vi "Main.vi"() -> ()   [LabVIEW 2017]
doc: "This VI was generated automatically using the FPGA Wizard. You can modify the VI normally."
uses:
  <vilib>/rvi/interface/nirviMethod/nirviMethod.xnode
  <vilib>/rvi/interface/nirviCloseFPGA/nirviCloseFPGA.xnode
  <vilib>/rvi/interface/nirviOpenFPGA/nirviOpenFPGA.xnode
  <vilib>/rvi/interface/nirviReadWriteControl/nirviReadWriteControl.xnode
  <vilib>/rvi/errors/niLvFpgaAdjustHostInterfaceError.vi
  <vilib>/rvi/interface/Simulation/niFpgaSimulationCallBeginRW.vi
  <vilib>/FPGAPlugInAG/Dynamic/niLvFpga_ReadFifo_Dynamic.vi
  <vilib>/rvi/errors/niLvFpgaMergeErrorWithErrorCode.vi
  HostCode.lvlib
  <vilib>/Utility/file.llb/Write To Spreadsheet File (I64).vi
  <vilib>/Utility/error.llb/Error Cluster From Error Code.vi
  NiFpgaLv.dll
  SerialComm/SerialComm.lvclass
  C:/Program Files (x86)/National Instruments/LabVIEW 2017/examples/Instrument IO/Serial/support/Serial - Settings.ctl
  <vilib>/FPGAPlugInAG/Dynamic/niLvFpga_Reset_Dynamic.vi
  <vilib>/FPGAPlugInAG/Dynamic/niLvFpga_Run_Dynamic.vi
  FPGA Bitfiles/ECGPWMAdaptiveFi_FPGATarget2_ECGAFSPIInput_AXfYGaptw90old.lvbitx
  <vilib>/FPGAPlugInAG/Dynamic/niLvFpga_Close_Dynamic.vi
  <vilib>/FPGAPlugInAG/USB-7856R/niLvFpga_Open_USB-7856R.vi
  <vilib>/rvi/interface/common/dynamic/niFpgaDynamicAddResources.vi
  FPGACode/Lead Enum.ctl
  Trigger Params.ctl
  FPGACode/Channel Enum.ctl
panel:
  in  "Beta":u8(slide)=1 scale=0.0..3.0
  in  "Sensis\nECG Scaling":i16=1 caption="ECG Output\nScaling" min=1 max=100 step=1
  in  "Tab Control":enum32{"Main", "Utilities"}(tab)
  out "ECG":i16[][](graph)
  out "Invasive Blood Pressure":i16[][](graph)
  in  "Trigger 2":T1={"Channel"=enum."II", "Threshold"=1000, "d/dt"=FALSE, "Invert"=FALSE}
  out "Trigger":i16[][](graph)
  in  "IBP Scale":fxp<+/-,16,5>=1.06005859375
  in  "IBP Offset":fxp<+/-,16,16>
  in  "IBP Filter":bool
  in  "ECG Filter":bool=TRUE
  in  "Plot Info":T4={"Element"={"Lead"=enum."I", "Filter"=TRUE}, "Element 2"={"Lead"=enum."II", "Filter"=TRUE}, "Element 3"={"Lead"=enum."III", "Filter"=TRUE}}
  out "Pressure Data":T5(array[cluster])
  out "Gradients":i16[][](graph)
  in  "Offset":cluster{"X":i16, "Y":i16, "Z":i16} {"Z" format="%.2f"; "Y" format="%.2f"; "X" format="%.2f"}
  in  "High Pass Filter":bool
  out "Taps":dbl[](graph)
  out "Weights":dbl[](graph)
  out "Beta Product":fxp<+/-,32,-1> format="%.3e"
  out "Weighted Sum":fxp<+/-,33,19> format="%.3e"
  in  "Channel":i32
  in  "ECG Input\nGain":u16(ring)=1 items=["1"=1, "2"=2, "3"=3, "4"=4, "6"=0, "8"=5, "12"=6]
  in  "ECG Beta":fxp<+/-,32,-16>=1.000088900582341e-11 format="%.3e"
  in  "Filter Size":i16=100
  in  "IBP Beta":fxp<+/-,32,-16> format="%.3e"
  in  "Record":bool
  in  "Path":path
  out "Loop Time":u32
  in  "Reset":bool
  out "Actual Loop Rate (Ticks)":u32
  out "Late? Latched":bool
  in  "Start":bool
  in  "Loop Rate (Hz)":dbl=10000.0
  out "Calculated Rate (Hz)":dbl
  out "error out":errorcluster
  in  "Global Stop":bool
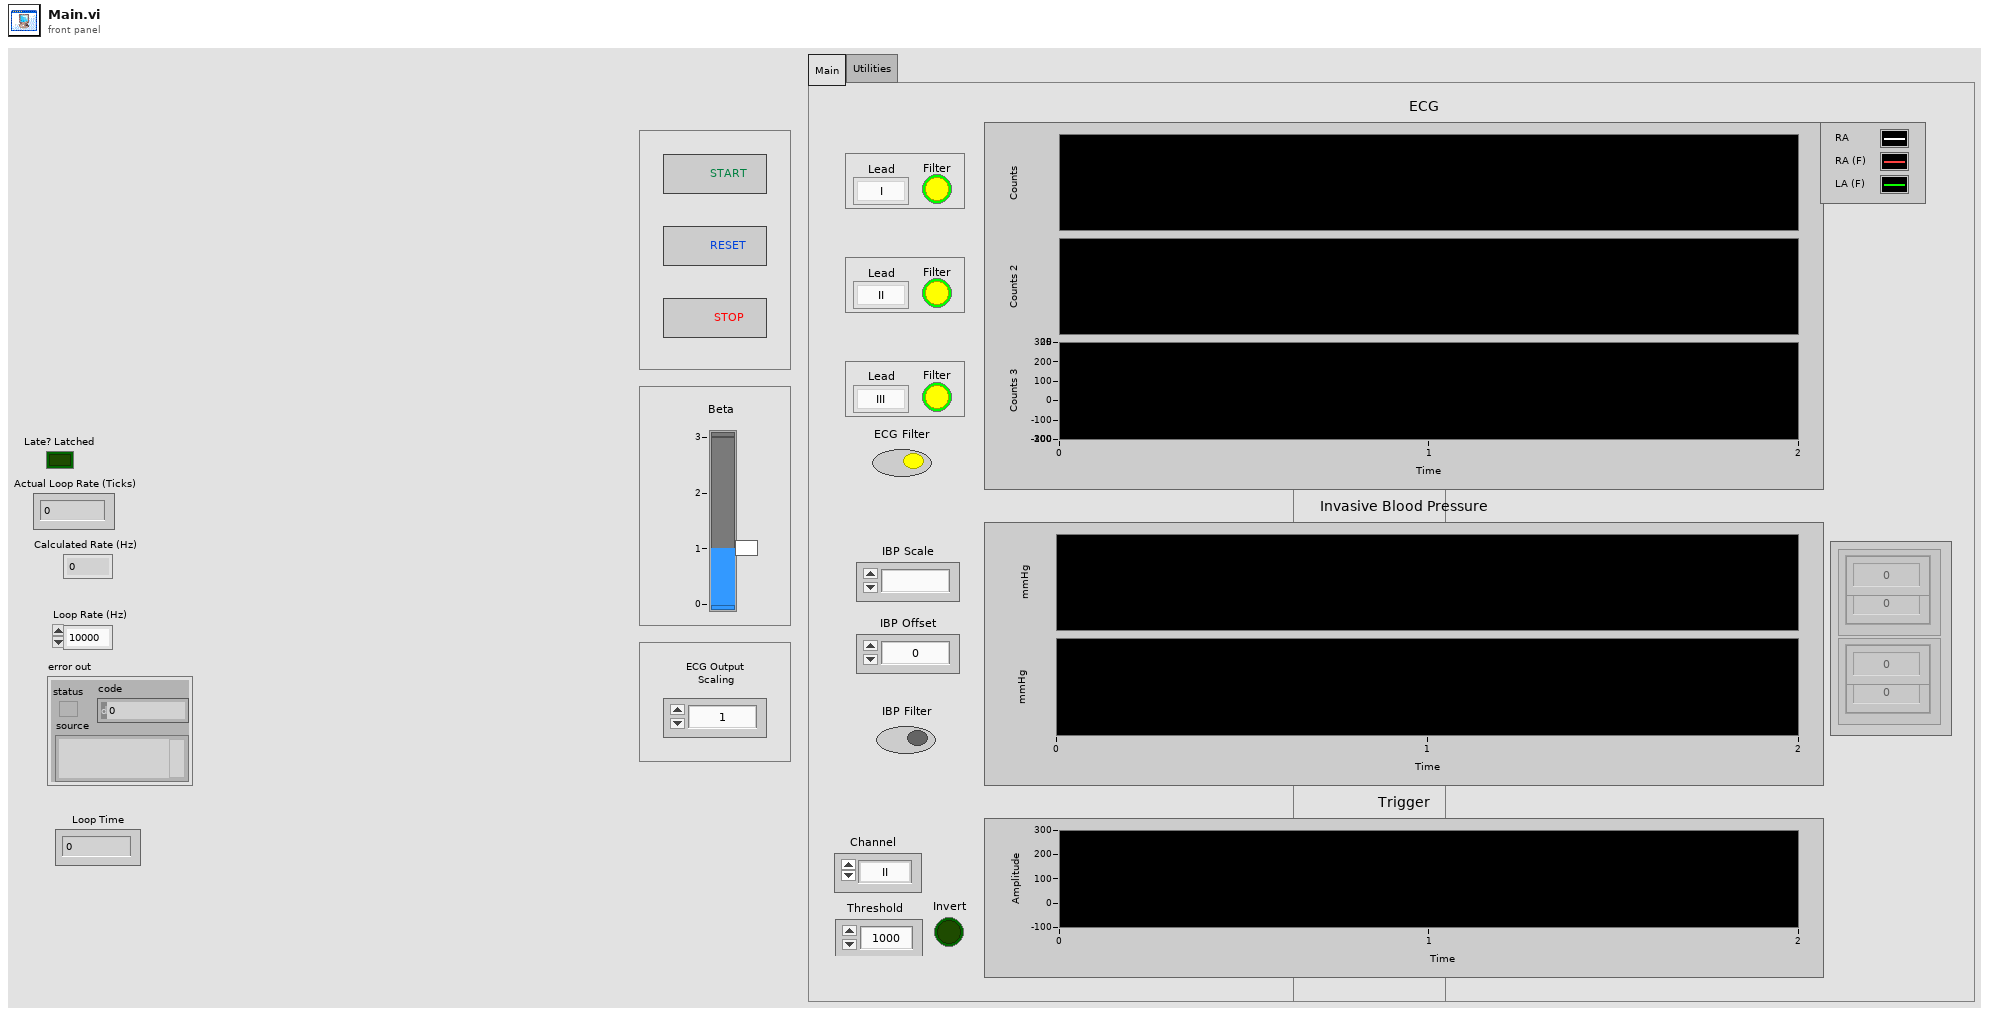
[diagram p1: front panel]
types:
  T1 = typedef "HostCode.lvlib/Trigger Params.ctl" = cluster{"Channel":T2, "Threshold":i16, "d/dt":bool, "Invert":bool}
  T2 = typedef "Channel Enum.ctl" = enum16{"RA", "LA", "LL", "V1", "V2", "V3", "V4", "V5", "V6", "I", "II", "III", "aVR", "aVL", "aVF", "Vw", "IBP1", "IBP2"}
  T3 = typedef "Lead Enum.ctl" = enum16{"RA", "LA", "LL", "V1", "V2", "V3", "V4", "V5", "V6", "I", "II", "III", "aVR", "aVL", "aVF", "Vw"}
  T4 = cluster{"Element":cluster{"Lead":T3, "Filter":bool}, "Element 2":cluster{"Lead":T3, "Filter":bool}, "Element 3":cluster{"Lead":T3, "Filter":bool}}
  T5 = cluster{"Numeric Control":dbl, "Numeric Control":dbl}[]
  T6 = typedef "Serial - Settings.ctl" = cluster{"baud rate":u32, "data bits":u16, "parity":enum16{"None", "Odd", "Even", "Mark", "Space"}, "stop bits":u16, "flow control":u16}
  T7 = enum8{"Enabled", "Disabled", "Disabled and Grayed Out"}
  T8 = typedef "LVOffsetAndMultiplierTypeDef.ctl" = cluster{"Offset":dbl, "Multiplier":dbl}
  T9 = cluster{"Channel":T2, "Threshold":i16, "Invert":bool}
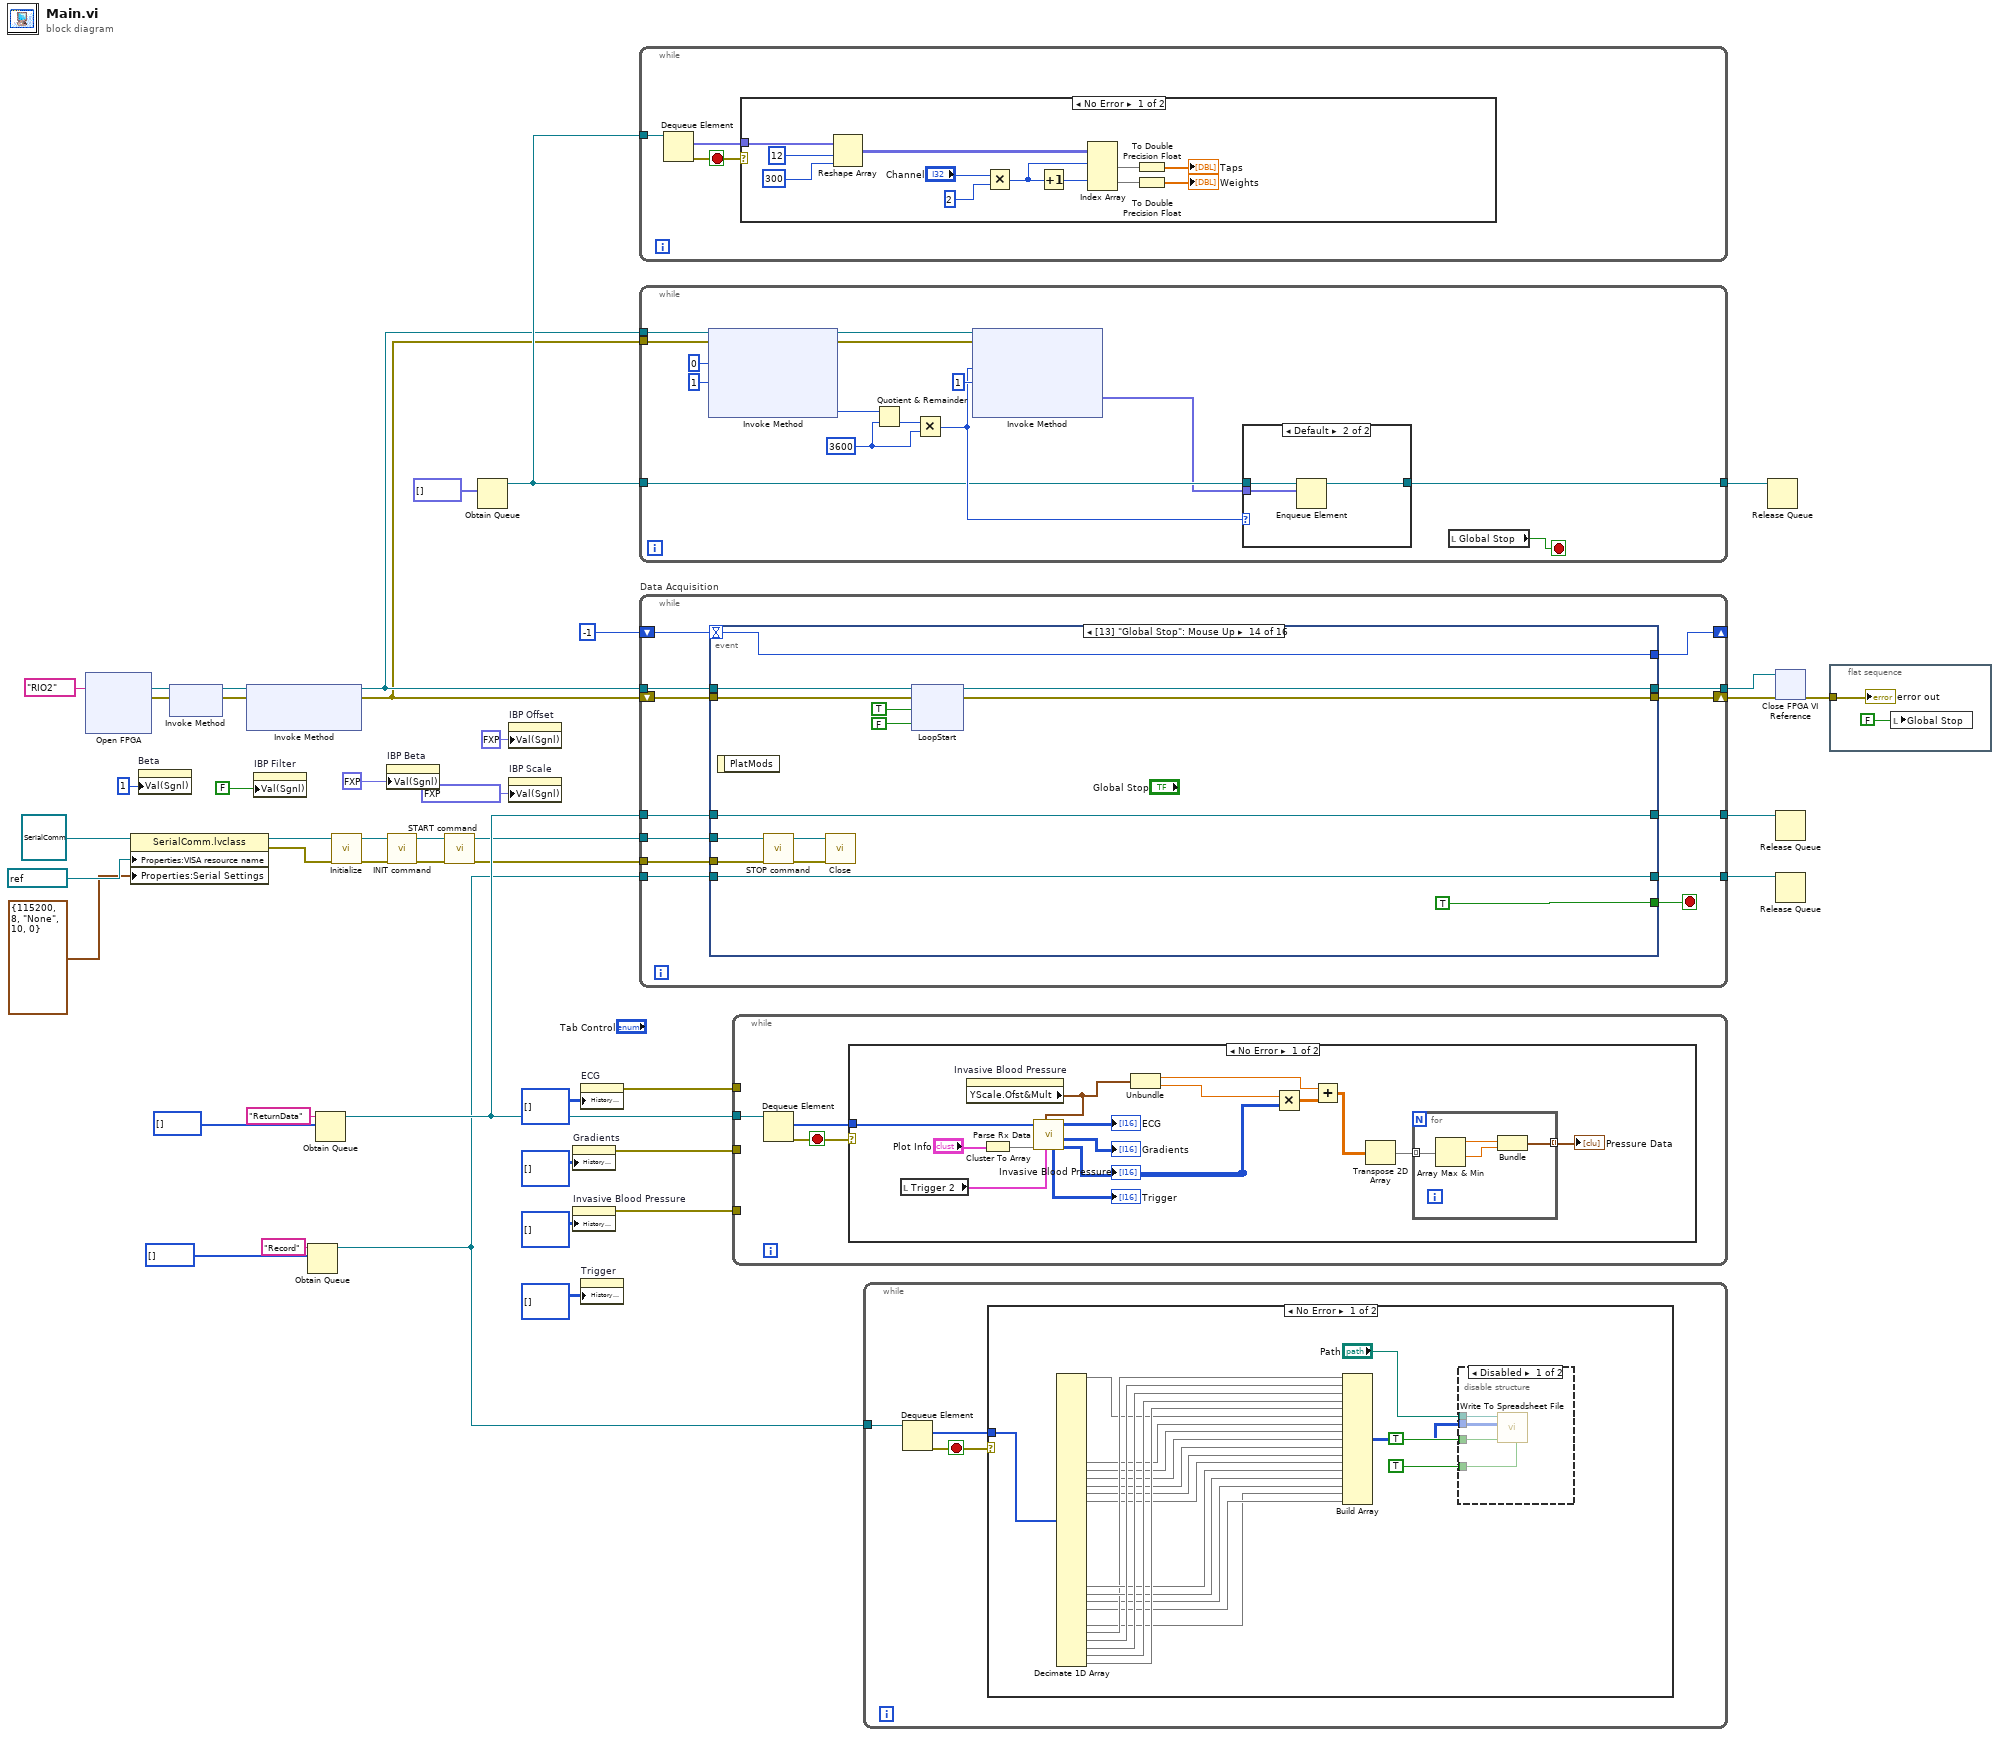
[diagram p0: block diagram]
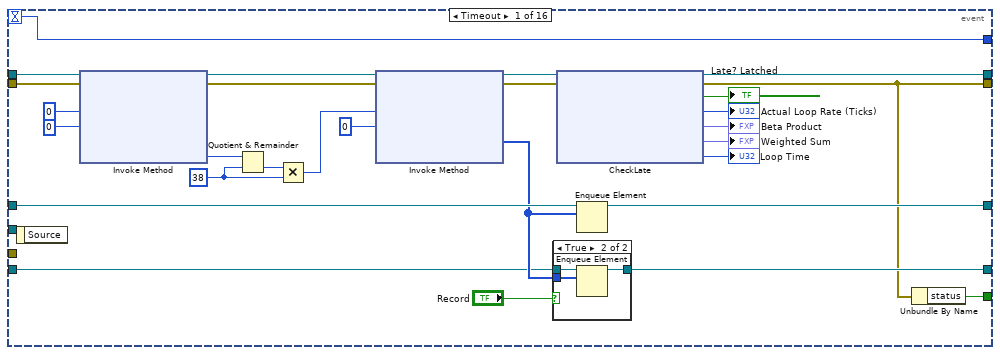
[diagram p2: hidden frame]
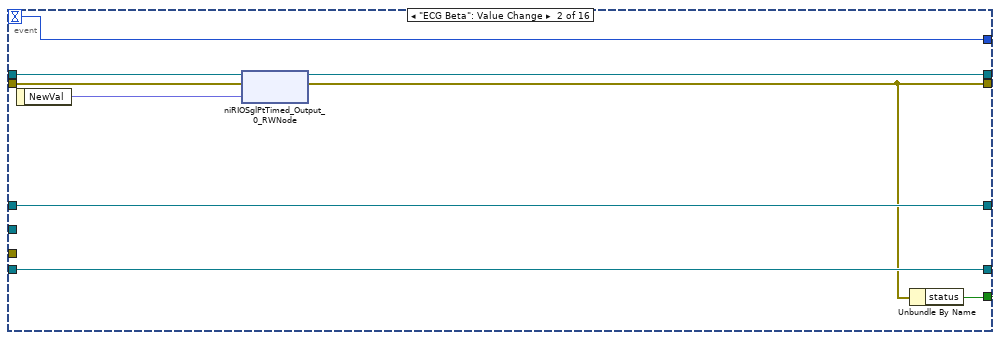
[diagram p4: hidden frame]
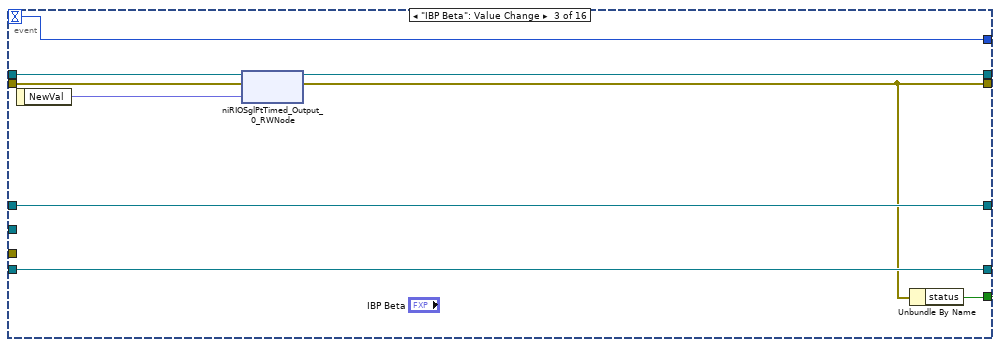
[diagram p5: hidden frame]
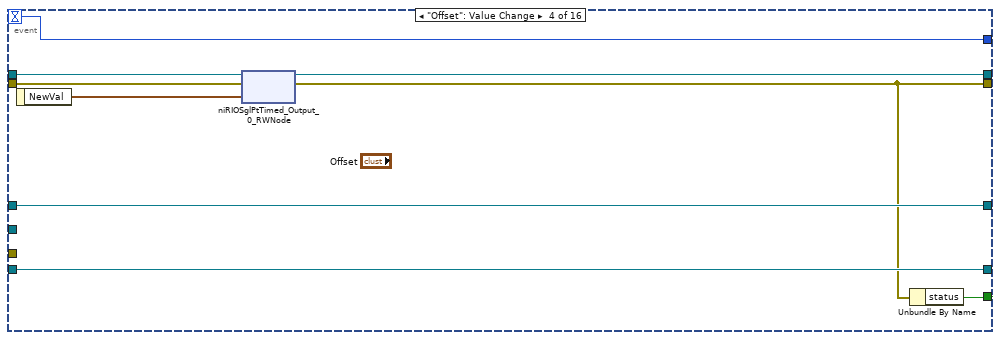
[diagram p6: hidden frame]
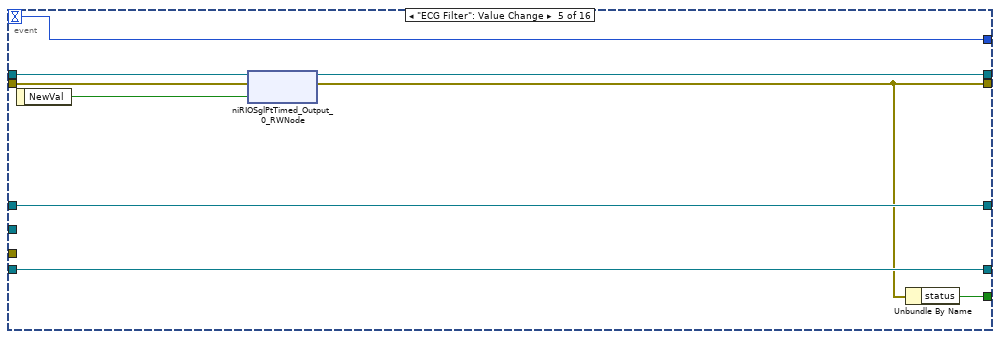
[diagram p7: hidden frame]
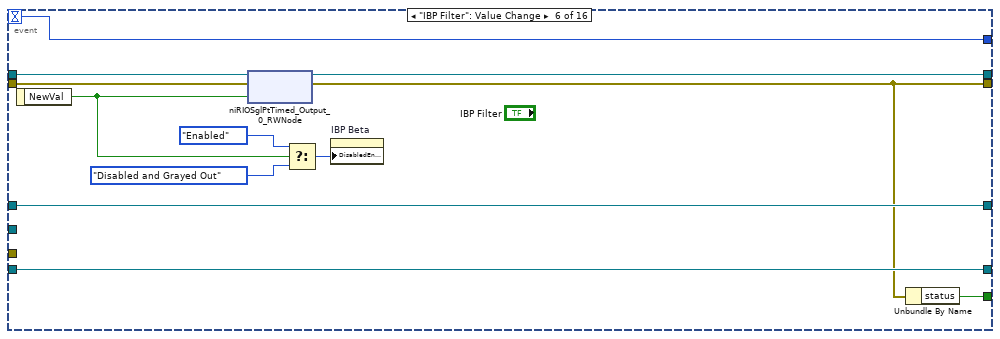
[diagram p8: hidden frame]
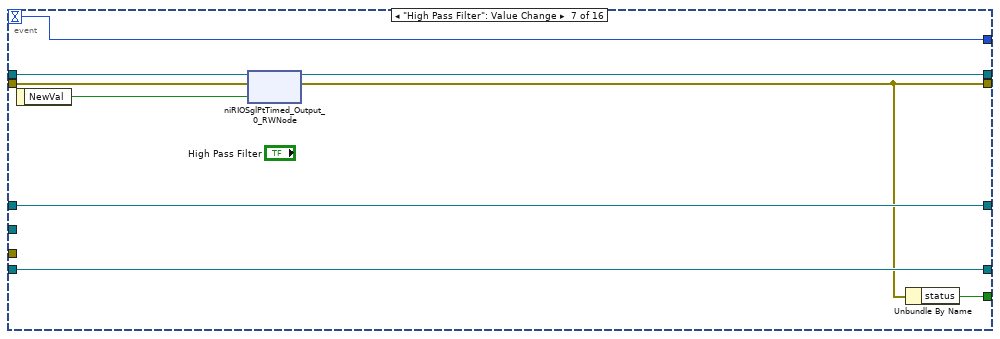
[diagram p9: hidden frame]
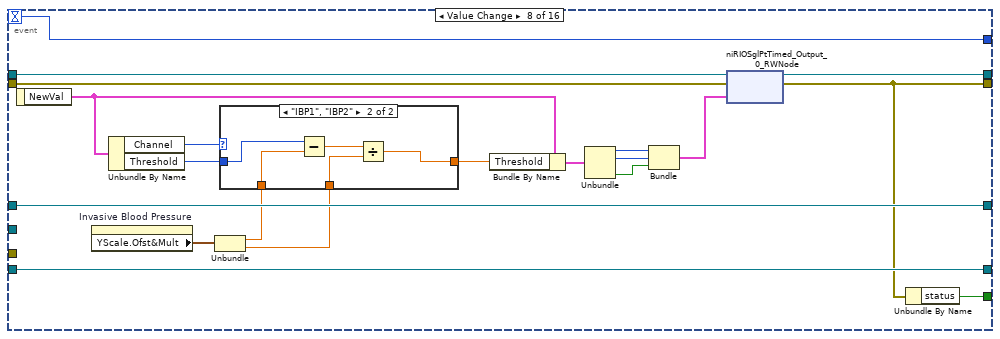
[diagram p10: hidden frame]
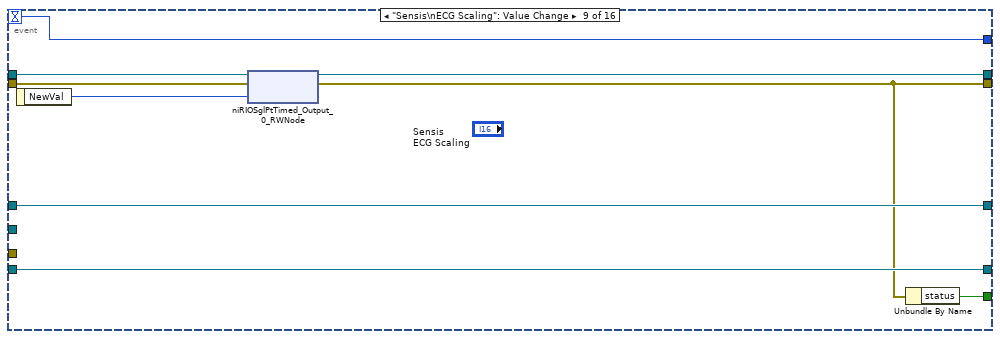
[diagram p12: hidden frame]
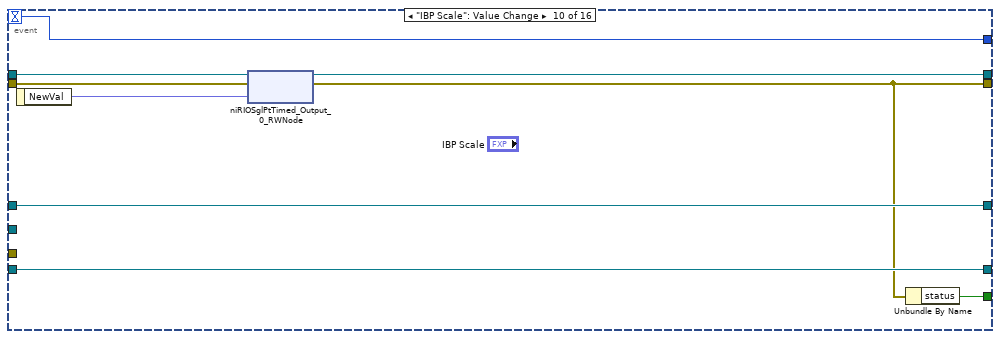
[diagram p13: hidden frame]
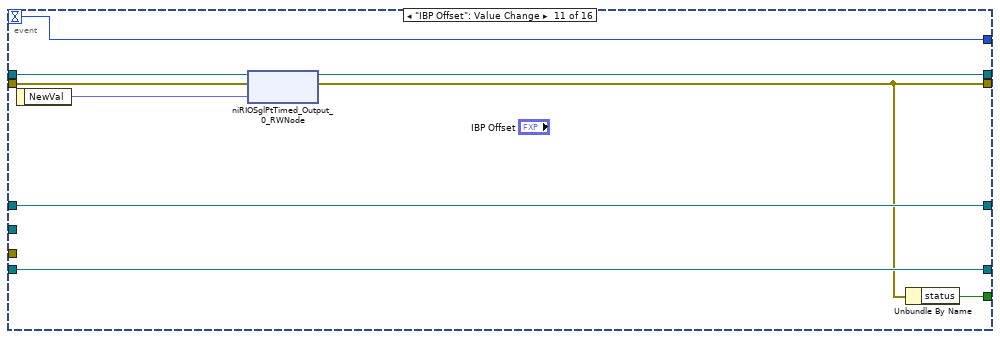
[diagram p14: hidden frame]
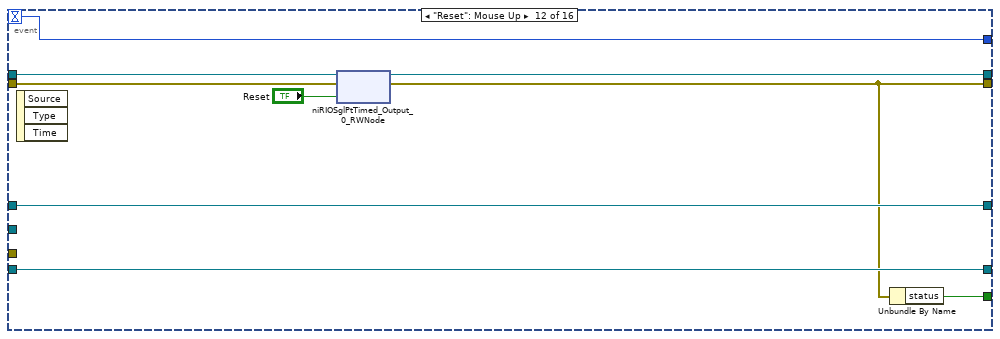
[diagram p15: hidden frame]
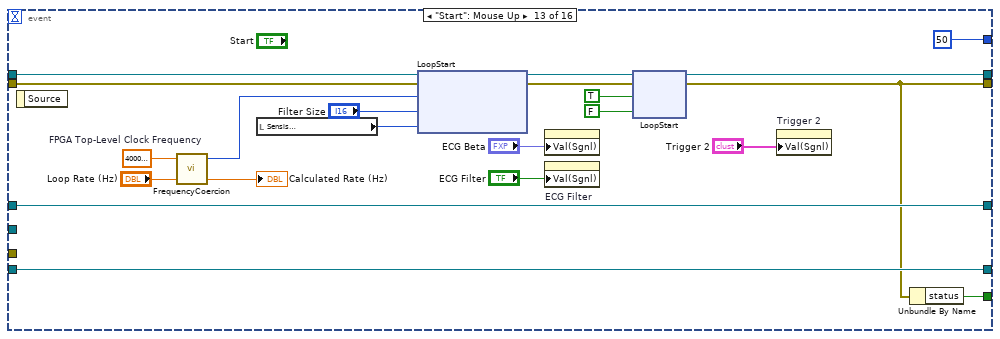
[diagram p16: hidden frame]
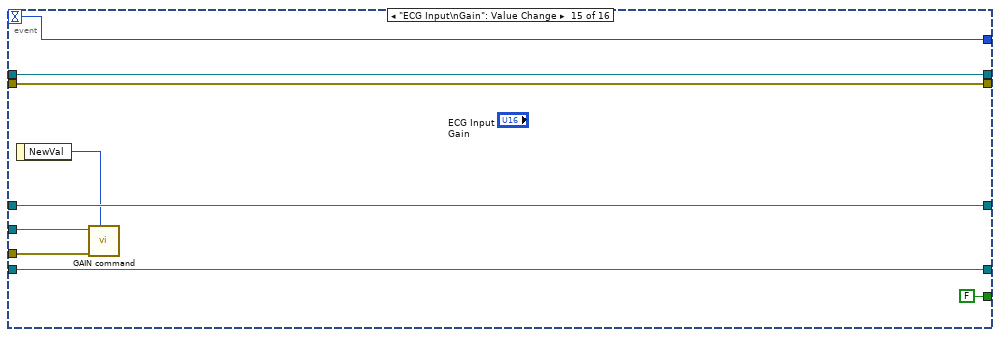
[diagram p17: hidden frame]
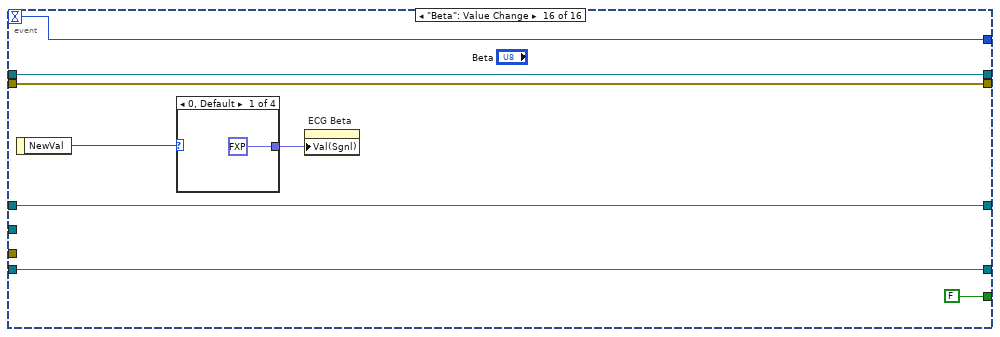
[diagram p18: hidden frame]
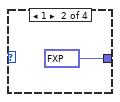
[diagram p19: hidden frame]
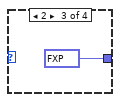
[diagram p20: hidden frame]
diagram:
  n1 = xnode ("Open FPGA")("resource name"=tag "RIO2") -> ("FPGA VI Reference Out"=w44:refnum<k20>, "error out"=w43:errorcluster)  [unwired: 1 in]
  n2 = property class="SerialComm.lvclass"(reference=refnum<class "SerialComm.lvclass"> refnum ("SerialComm.lvclass"), "Properties:VISA resource name"=refnum<visa-resource-name> "COM4" ("VISA resource name"), "Properties:Serial Settings"=T6 {"baud rate"=115200, "data bits"=8, "parity"=enum."None", "stop bits"=10, "flow control"=0} ("Serial Settings")) -> (reference out=w13:refnum<class "SerialComm.lvclass">, error out=w9:errorcluster)  [unwired: 1 in]
  n3 = property on="Beta" class="Slide (strict)"("Val(Sgnl)"=u8 1 ("Value (Signaling)")) -> ()  [unwired: 2 in, 2 out]
  n4 = xnode ("Invoke Method")("FPGA VI Reference In"=w44, "error in"=w43) -> ("FPGA VI Reference Out"=w21:refnum<k20>, "error out"=w45:errorcluster)
  n5 = xnode ("Invoke Method")("FPGA VI Reference In"=w21, "error in"=w45) -> ("FPGA VI Reference Out"=w19:refnum<k20>, "error out"=w18:errorcluster)  [unwired: 1 in]
  n6 = property on="IBP Filter" class="Bool (strict)"("Val(Sgnl)"=FALSE ("Value (Signaling)")) -> ()  [unwired: 2 in, 2 out]
  n7 = Obtain Queue(name (unnamed)="Record", element data type=i16[] []) -> (queue out=w29:refnum<queue>)  [unwired: 3 in, 2 out]
  n8 = Obtain Queue(name (unnamed)="ReturnData", element data type=i16[] []) -> (queue out=w37:refnum<queue>)  [unwired: 3 in, 2 out]
  n9 = call "Initialize.vi"("Error In"=w9, "SerialComm in"=w13) -> ("Error Out"=w8:errorcluster, "SerialComm out"=w12:refnum<class "SerialComm.lvclass">)  [unwired: 8 in]
  n10 = property on="IBP Beta" class="DigNum (strict)"("Val(Sgnl)"=fxp<+/-,32,-16> 0.0 ("Value (Signaling)")) -> ()  [unwired: 2 in, 2 out]
  n11 = call "INIT command.vi"("Error In"=w8, "SerialComm in"=w12) -> ("Error Out"=w7:errorcluster, "SerialComm out"=w11:refnum<class "SerialComm.lvclass">)  [unwired: 8 in]
  n12 = call "START command.vi"("Error In"=w7, "SerialComm in"=w11) -> ("Error Out"=w6:errorcluster, "SerialComm out"=w10:refnum<class "SerialComm.lvclass">)  [unwired: 8 in]
  n13 = Obtain Queue(element data type=fxp<+/-,32,16>[] [] ("Data")) -> (queue out=w24:refnum<queue>)  [unwired: 4 in, 2 out]
  n14 = property on="IBP Offset" class="DigNum (strict)"("Val(Sgnl)"=fxp<+/-,16,16> 0.0 ("Value (Signaling)")) -> ()  [unwired: 2 in, 2 out]
  n15 = property on="IBP Scale" class="DigNum (strict)"("Val(Sgnl)"=fxp<+/-,16,5> 1.06005859375 ("Value (Signaling)")) -> ()  [unwired: 2 in, 2 out]
  n16 = property on="Gradients" class="WFChart (strict)"("History Data"=i16[][] []) -> (error out=w34:errorcluster)  [unwired: 2 in, 1 out]
  n17 = property on="Invasive Blood Pressure" class="WFChart (strict)"("History Data"=i16[][] []) -> (error out=w26:errorcluster)  [unwired: 2 in, 1 out]
  n18 = property on="ECG" class="WFChart (strict)"("History Data"=i16[][] []) -> (error out=w35:errorcluster)  [unwired: 2 in, 1 out]
  n19 = property on="Trigger" class="WFChart (strict)"("History Data"=i16[][] []) -> ()  [unwired: 2 in, 2 out]
  n20 = while {
    tunnel: w24 -> [w48]
    stop <- w46 stop-if-true
    n21 = Dequeue Element(queue=w48) -> (element=w47:fxp<+/-,32,16>[], error out=w46:errorcluster)  [unwired: 2 in, 2 out]
    n22 = case shown="No Error" w46 {
      tunnel: w47 -> [w60 _]
      frame No Error {
        n23 = Reshape Array(w60, 12 ("dimension size"), 300 ("dimension size")) -> (w56:fxp<+/-,32,16>[][])
        n24 = Multiply(x="Channel", y=2) -> (x*y=w49:i32)
        n25 = Increment(x=w49) -> (x+1=w50:i32)
        n26 = Index Array(array=w56, index (row) #1=w49, index (row) #2=w50) -> (element #1=w55:fxp<+/-,32,16>[], element #2=w54:fxp<+/-,32,16>[])  [unwired: 2 in]
        n27 = To Double Precision Float(number=w55) -> (double precision float=→"Taps":dbl[])
        n28 = To Double Precision Float(number=w54) -> (double precision float=→"Weights":dbl[])
      }
      frame Error {
      }
    }
  }
  n29 = while {
    tunnel: w19 -> [w75]
    tunnel: w18 -> [w74]
    tunnel: w24 -> [w63]
    tunnel: [w61] -> w23
    stop <- w66 stop-if-true
    w68 = u32 3600 ("y")
    n30 = xnode "Invoke Method"("FPGA VI Reference In"=w75, "error in"=w74, "Number of Elements"=u32 0, "Timeout (ms)"=1) -> ("FPGA VI Reference Out"=w71:refnum<k20>, "error out"=w70:errorcluster, "Elements Remaining"=w67:u32)  [unwired: 1 out]
    n31 = Quotient & Remainder(x=w67, y=w68) -> (floor(x/y)=w69:u32)  [unwired: 1 out]
    n32 = Multiply(x=w69, y=w68) -> (x*y=w64:u32)
    n33 = xnode "Invoke Method"("FPGA VI Reference In"=w71, "error in"=w70, "Number of Elements"=w64, "Timeout (ms)"=1) -> ("Data"=w62:fxp<+/-,32,16>[])  [unwired: 3 out]
    n34 = case shown="Default" w64 {
      tunnel: w63 -> [w76 w79]
      tunnel: w62 -> [_ w78]
      tunnel: [w76 w77] -> w61
      frame 0 {
      }
      frame Default {
        n35 = Enqueue Element(queue=w79, element=w78) -> (queue out=w77:refnum<queue>)  [unwired: 2 in, 2 out]
      }
    }
    n36 = local read "Global Stop"() -> (w66:bool)
  }
  n37 = while "Data Acquisition" {
    tunnel: w19 -> [w88]
    shift-right: [w92] -> w42
    shift-left: w18 -> [w89]
    tunnel: [w90] -> w40
    tunnel: w37 -> [w87]
    tunnel: [w86] -> w32
    tunnel: w29 -> [w85]
    tunnel: [w84] -> w28
    shift-right: [w82] -> _
    shift-left: -1 -> [w83]
    tunnel: w10 -> [w81]
    tunnel: w6 -> [w80]
    stop <- w91 stop-if-true
    n38 = event shown="[13] \"Global Stop\": Mouse Up" {
      selector: _ -> [_ _ _ _ _ _ _ _ _ _ _ _ _ _ _ _]
      dyn-events: _ -> [_ _ _ _ _ _ _ _ _ _ _ _ _ _ _ _]
      timeout: w83 -> [w95 w127 w136 w145 w154 w167 w175 w196 w211 w220 w229 w237 _ w271 w285 w294]
      tunnel: [w94 w126 w135 w144 w153 w166 w174 w195 w210 w219 w228 w236 w247 w272 w286 w293] -> w92
      tunnel: [w93 w125 w134 w143 w152 w165 w173 w194 w209 w218 w227 w235 w246 TRUE FALSE ("status") FALSE ("status")] -> w91
      tunnel: [w120 w131 w140 w149 w158 w170 w179 w199 w214 w223 w232 w241 w252 w273 w287 w295] -> w90
      tunnel: w89 -> [w97 w132 w141 w150 w159 w171 w180 w200 w215 w224 w233 w242 w262 w274 w286 w293]
      tunnel: w88 -> [w98 w133 w142 w151 w160 w172 w181 w201 w216 w225 w234 w243 w263 w275 w287 w295]
      tunnel: w87 -> [w109 w129 w138 w147 w156 w169 w177 w198 w213 w222 w231 w240 w261 w278 w284 w292]
      tunnel: [w105 w129 w138 w147 w156 w169 w177 w198 w213 w222 w231 w240 w261 w278 w284 w292] -> w86
      tunnel: w85 -> [w102 w128 w137 w146 w155 w168 w176 w197 w212 w221 w230 w239 w260 w277 w283 w291]
      tunnel: [w96 w128 w137 w146 w155 w168 w176 w197 w212 w221 w230 w239 w260 w277 w283 w291] -> w84
      tunnel: [w95 w127 w136 w145 w154 w167 w175 w196 w211 w220 w229 w237 50 w271 w285 w294] -> w82
      tunnel: w81 -> [_ _ _ _ _ _ _ _ _ _ _ _ _ w268 w281 _]
      tunnel: w80 -> [_ _ _ _ _ _ _ _ _ _ _ _ _ w267 w280 _]
      event Timeout {
        w107 = u32 38 ("y")
        n39 = event-data() -> ()  [unwired: 1 in, 1 out]
        n40 = xnode "Invoke Method"("FPGA VI Reference In"=w98, "error in"=w97, "Number of Elements"=u32 0, "Timeout (ms)"=0) -> ("FPGA VI Reference Out"=w115:refnum<k20>, "error out"=w114:errorcluster, "Elements Remaining"=w113:u32)  [unwired: 1 out]
        n41 = Quotient & Remainder(x=w113, y=w107) -> (floor(x/y)=w108:u32)  [unwired: 1 out]
        n42 = Multiply(x=w108, y=w107) -> (x*y=w106:u32)
        n43 = xnode "Invoke Method"("FPGA VI Reference In"=w115, "error in"=w114, "Number of Elements"=w106, "Timeout (ms)"=0) -> ("FPGA VI Reference Out"=w111:refnum<k20>, "error out"=w110:errorcluster, "Data"=w103:i16[])  [unwired: 1 out]
        n44 = case shown="True" "Record" {
          tunnel: w103 -> [_ w124]
          tunnel: w102 -> [w121 w123]
          tunnel: [w121 w122] -> w96
          frame False {
          }
          frame True {
            n45 = Enqueue Element(queue=w123, element=w124) -> (queue out=w122:refnum<queue>)  [unwired: 2 in, 2 out]
          }
        }
        n46 = xnode ("CheckLate")("FPGA VI Reference In"=w111, "error in"=w110) -> ("FPGA VI Reference Out"=w120:refnum<k20>, "error out"=w94:errorcluster, "Late? Latched"=→"Late? Latched":bool, "Actual Loop Rate (Ticks)"=→"Actual Loop Rate (Ticks)":u32, "BetaProduct"=→"Beta Product":fxp<+/-,32,-1>, "WeightSum"=→"Weighted Sum":fxp<+/-,33,19>, "Loop Time"=→"Loop Time":u32)
        n47 = Enqueue Element(queue=w109, element=w103) -> (queue out=w105:refnum<queue>)  [unwired: 2 in, 2 out]
        n48 = Unbundle By Name(w94) -> ("status"=w93:bool)
      }
      event "ECG Beta": Value Change {
        n49 = event-data() -> ("NewVal"=w130:fxp<+/-,32,-16>)  [unwired: 1 in]
        n50 = xnode ("niRIOSglPtTimed_Output_0_RWNode")("FPGA VI Reference In"=w133, "error in"=w132, "Beta ECG"=w130) -> ("FPGA VI Reference Out"=w131:refnum<k20>, "error out"=w126:errorcluster)
        n51 = Unbundle By Name(w126) -> ("status"=w125:bool)
      }
      event "IBP Beta": Value Change {
        n52 = event-data() -> ("NewVal"=w139:fxp<+/-,32,-16>)  [unwired: 1 in]
        n53 = xnode ("niRIOSglPtTimed_Output_0_RWNode")("FPGA VI Reference In"=w142, "error in"=w141, "Beta IBP"=w139) -> ("FPGA VI Reference Out"=w140:refnum<k20>, "error out"=w135:errorcluster)
        n54 = Unbundle By Name(w135) -> ("status"=w134:bool)
      }
      event "Offset": Value Change {
        n55 = event-data() -> ("NewVal"=w148:cluster{"X":i16, "Y":i16, "Z":i16})  [unwired: 1 in]
        n56 = xnode ("niRIOSglPtTimed_Output_0_RWNode")("FPGA VI Reference In"=w151, "error in"=w150, "Offset"=w148) -> ("FPGA VI Reference Out"=w149:refnum<k20>, "error out"=w144:errorcluster)
        n57 = Unbundle By Name(w144) -> ("status"=w143:bool)
      }
      event "ECG Filter": Value Change {
        n58 = event-data() -> ("NewVal"=w157:bool)  [unwired: 1 in]
        n59 = xnode ("niRIOSglPtTimed_Output_0_RWNode")("FPGA VI Reference In"=w160, "error in"=w159, "ECG Filter"=w157) -> ("FPGA VI Reference Out"=w158:refnum<k20>, "error out"=w153:errorcluster)
        n60 = Unbundle By Name(w153) -> ("status"=w152:bool)
      }
      event "IBP Filter": Value Change {
        n61 = event-data() -> ("NewVal"=w164:bool)  [unwired: 1 in]
        n62 = xnode ("niRIOSglPtTimed_Output_0_RWNode")("FPGA VI Reference In"=w172, "error in"=w171, "IBP Filter"=w164) -> ("FPGA VI Reference Out"=w170:refnum<k20>, "error out"=w166:errorcluster)
        n63 = Select(t=T7."Enabled" ("Disabled"), s=w164, f=T7."Disabled and Grayed Out" ("Disabled")) -> (s? t:f=w161:T7)
        n64 = property on="IBP Beta" class="DigNum (strict)"("DisabledEnum"=w161) -> ()  [unwired: 2 in, 2 out]
        n65 = Unbundle By Name(w166) -> ("status"=w165:bool)
      }
      event "High Pass Filter": Value Change {
        n66 = event-data() -> ("NewVal"=w178:bool)  [unwired: 1 in]
        n67 = xnode ("niRIOSglPtTimed_Output_0_RWNode")("FPGA VI Reference In"=w181, "error in"=w180, "HPF"=w178) -> ("FPGA VI Reference Out"=w179:refnum<k20>, "error out"=w174:errorcluster)
        n68 = Unbundle By Name(w174) -> ("status"=w173:bool)
      }
      event Value Change {
        n69 = event-data() -> ("NewVal"=w191:T1)  [unwired: 1 in]
        n70 = property on="Invasive Blood Pressure" class="WFChart (strict)"() -> ("YScale.Ofst&Mult"=w189:T8)  [unwired: 2 in, 2 out]
        n71 = Unbundle By Name(w191) -> ("Channel"=w193:T2, "Threshold"=w192:i16)
        n72 = Unbundle(w189) -> ("Offset"=w188:dbl, "Multiplier"=w187:dbl)
        n73 = case shown="\"IBP1\", \"IBP2\"" w193 {
          tunnel: w192 -> [w202 w207]
          tunnel: [w202 w203] -> w190
          tunnel: w188 -> [_ w206]
          tunnel: w187 -> [_ w204]
          frame Default {
          }
          frame "IBP1", "IBP2" {
            n74 = Subtract(x=w207, y=w206) -> (x-y=w205:dbl)
            n75 = Divide(x=w205, y=w204) -> (x/y=w203:dbl)
          }
        }
        n76 = Bundle By Name(cluster=w191, "Threshold"=w190) -> (w186:T1)
        n77 = Unbundle(w186) -> ("Channel"=w185:T2, "Threshold"=w184:i16, "Invert"=w183:bool)  [unwired: 1 out]
        n78 = Bundle("Channel"=w185, "Threshold"=w184, "Invert"=w183) -> (w182:T9)  [unwired: 1 in]
        n79 = xnode ("niRIOSglPtTimed_Output_0_RWNode")("FPGA VI Reference In"=w201, "error in"=w200, "Trigger"=w182) -> ("FPGA VI Reference Out"=w199:refnum<k20>, "error out"=w195:errorcluster)
        n80 = Unbundle By Name(w195) -> ("status"=w194:bool)
      }
      event "Sensis\nECG Scaling": Value Change {
        n81 = event-data() -> ("NewVal"=w208:i16)  [unwired: 1 in]
        n82 = xnode ("niRIOSglPtTimed_Output_0_RWNode")("FPGA VI Reference In"=w216, "error in"=w215, "ECG Scale"=w208) -> ("FPGA VI Reference Out"=w214:refnum<k20>, "error out"=w210:errorcluster)
        n83 = Unbundle By Name(w210) -> ("status"=w209:bool)
      }
      event "IBP Scale": Value Change {
        n84 = event-data() -> ("NewVal"=w217:fxp<+/-,16,5>)  [unwired: 1 in]
        n85 = xnode ("niRIOSglPtTimed_Output_0_RWNode")("FPGA VI Reference In"=w225, "error in"=w224, "IBP Scale"=w217) -> ("FPGA VI Reference Out"=w223:refnum<k20>, "error out"=w219:errorcluster)
        n86 = Unbundle By Name(w219) -> ("status"=w218:bool)
      }
      event "IBP Offset": Value Change {
        n87 = event-data() -> ("NewVal"=w226:fxp<+/-,16,16>)  [unwired: 1 in]
        n88 = xnode ("niRIOSglPtTimed_Output_0_RWNode")("FPGA VI Reference In"=w234, "error in"=w233, "IBP Offset"=w226) -> ("FPGA VI Reference Out"=w232:refnum<k20>, "error out"=w228:errorcluster)
        n89 = Unbundle By Name(w228) -> ("status"=w227:bool)
      }
      event "Reset": Mouse Up {
        n90 = event-data() -> ()  [unwired: 1 in, 3 out]
        n91 = xnode ("niRIOSglPtTimed_Output_0_RWNode")("FPGA VI Reference In"=w243, "error in"=w242, "Reset"="Reset") -> ("FPGA VI Reference Out"=w241:refnum<k20>, "error out"=w236:errorcluster)
        n92 = Unbundle By Name(w236) -> ("status"=w235:bool)
      }
      event "Start": Mouse Up {
        w259 = 40000000.0  # FPGA Top-Level Clock Frequency
        n93 = event-data() -> ()  [unwired: 1 in, 1 out]
        n94 = call "FrequencyCoercion.vi"("Loop Rate (Hz)"="Loop Rate (Hz)", "FPGA Top-Level Clock Frequency"=w259) -> ("Actual Rate (Hz)"=→"Calculated Rate (Hz)":dbl, "FPGA Ticks"=w256:u32)  [unwired: 2 in]
        n95 = local read "Sensis\nECG Scaling"() -> (w244:i16)
        n96 = xnode ("LoopStart")("FPGA VI Reference In"=w263, "error in"=w262, "Loop Rate (Ticks)"=w256, "Filter Size"="Filter Size", "ECG Scale"=w244) -> ("FPGA VI Reference Out"=w254:refnum<k20>, "error out"=w253:errorcluster)
        n97 = property on="ECG Beta" class="DigNum (strict)"("Val(Sgnl)"="ECG Beta") -> ()  [unwired: 2 in, 2 out]
        n98 = property on="ECG Filter" class="Bool (strict)"("Val(Sgnl)"="ECG Filter") -> ()  [unwired: 2 in, 2 out]
        n99 = xnode ("LoopStart")("FPGA VI Reference In"=w254, "error in"=w253, "Start"=TRUE ("Start 0"), "Start"=FALSE ("Start 0")) -> ("FPGA VI Reference Out"=w252:refnum<k20>, "error out"=w247:errorcluster)
        n100 = property on="Trigger 2" class="Clust (strict)"("Val(Sgnl)"="Trigger 2") -> ()  [unwired: 2 in, 2 out]
        n101 = Unbundle By Name(w247) -> ("status"=w246:bool)
      }
      event "Global Stop": Mouse Up {
        n102 = event-data() -> ()  [unwired: 1 in, 1 out]
        n103 = call "STOP command.vi"("Error In"=w267, "SerialComm in"=w268) -> ("Error Out"=w265:errorcluster, "SerialComm out"=w266:refnum<class "SerialComm.lvclass">)  [unwired: 8 in]
        n104 = call "Close.vi"("Error In"=w265, "SerialComm in"=w266) -> ()  [unwired: 8 in, 2 out]
        n105 = xnode ("LoopStart")("FPGA VI Reference In"=w275, "error in"=w274, "Stop"=TRUE ("stop"), "Stop"=FALSE ("stop")) -> ("FPGA VI Reference Out"=w273:refnum<k20>, "error out"=w272:errorcluster)
      }
      event "ECG Input\nGain": Value Change {
        n106 = event-data() -> ("NewVal"=w279:u16)  [unwired: 1 in]
        n107 = call "GAIN command.vi"("Ring"=w279, "Error In"=w280, "SerialComm in"=w281) -> ()  [unwired: 7 in, 2 out]
      }
      event "Beta": Value Change {
        n108 = event-data() -> ("NewVal"=w289:u8)  [unwired: 1 in]
        n109 = case shown="0, Default" w289 {
          tunnel: [fxp<+/-,32,-16> 0.0 ("Value (Signaling)") fxp<+/-,32,-16> 1.000088900582341e-11 ("Value (Signaling)") fxp<+/-,32,-16> 9.99982319171977e-11 ("Value (Signaling)") fxp<+/-,32,-16> 1.000000082740371e-09 ("Value (Signaling)")] -> w288
          frame 0, Default {
          }
          frame 1 {
          }
          frame 2 {
          }
          frame 3 {
          }
        }
        n110 = property on="ECG Beta" class="DigNum (strict)"("Val(Sgnl)"=w288) -> ()  [unwired: 2 in, 2 out]
      }
    }
  }
  n111 = while {
    tunnel: w37 -> [w302]
    tunnel: w35 -> [_]
    tunnel: w34 -> [_]
    tunnel: w26 -> [_]
    stop <- w301 stop-if-true
    n112 = Dequeue Element(queue=w302) -> (element=w300:i16[], error out=w301:errorcluster)  [unwired: 2 in, 2 out]
    n113 = case shown="No Error" w301 {
      tunnel: w300 -> [w317 _]
      frame No Error {
        n114 = local read "Trigger 2"() -> (w314:T1)
        n115 = property on="Invasive Blood Pressure" class="WFChart (strict)"() -> ("YScale.Ofst&Mult"=w303:T8)  [unwired: 2 in, 2 out]
        n116 = Cluster To Array(cluster="Plot Info") -> (array=w309:cluster{"Lead":T3, "Filter":bool}[])
        n117 = call "Parse Rx Data.vi"("Trigger"=w314, "Scale"=w303, "Plot Info"=w309, "Input Data"=w317) -> ("Pressures"=w305:i16[][], "Gradients"=→"Gradients":i16[][], "ECG Data"=→"ECG":i16[][], "Trigger"=→"Trigger":i16[][])  [unwired: 4 in]
        "Invasive Blood Pressure" <- w305
        n118 = Unbundle(w303) -> ("Offset"=w306:dbl, "Multiplier"=w308:dbl)
        n119 = Multiply(x=w308, y=w305) -> (x*y=w307:dbl[][])
        n120 = Add(x=w306, y=w307) -> (x+y=w304:dbl[][])
        n121 = Transpose 2D Array(2D array=w304) -> (transposed array=w310:dbl[][])
        n122 = for {
          tunnel: w310 -> [w321] mode=indexing
          tunnel: [w318] -> w311 mode=indexing
          n123 = Array Max & Min(array=w321) -> (max value=w320:dbl, min value=w319:dbl)  [unwired: 2 out]
          n124 = Bundle(w320, w319) -> (w318:cluster{dbl, dbl})  [unwired: 1 in]
        }
        "Pressure Data" <- w311
      }
      frame Error {
      }
    }
  }
  n125 = while {
    tunnel: w29 -> [w322]
    stop <- w324 stop-if-true
    n126 = Dequeue Element(queue=w322) -> (element=w323:i16[], error out=w324:errorcluster)  [unwired: 2 in, 2 out]
    n127 = case shown="No Error" w324 {
      tunnel: w323 -> [w343 _]
      frame No Error {
        n128 = Decimate 1D Array(w343) -> (w328:i16[], w334:i16[], w333:i16[], w332:i16[], w331:i16[], w330:i16[], w327:i16[], w337:i16[], w338:i16[], w326:i16[], w329:i16[], w325:i16[], w335:i16[], w342:i16[], w341:i16[], w340:i16[], w339:i16[])  [unwired: 21 out]
        n129 = Build Array(w335, w342, w341, w340, w339, w328, w334, w333, w332, w331, w330, w327, w337, w338, w326, w325, w329) -> (w336:i16[][])
        n130 = disable-structure shown="Disabled" {
          disable-tunnel: "Path" -> [w350 _]
          disable-tunnel: TRUE ("transpose? (no:F)") -> [w349 _]
          disable-tunnel: TRUE ("append to file? (new file:F)") -> [w348 _]
          disable-tunnel: w336 -> [w347 _]
          frame Disabled {
            n131 = call-poly <vilib>:"Write To Spreadsheet File.vi"("transpose? (no:F)"=w349, "append to file? (new file:F)"=w348, "2D data"=w347, "file path (dialog if empty)"=w350) -> ()  [unwired: 4 in, 1 out]
          }
          frame Enabled {
          }
        }
      }
      frame Error {
      }
    }
  }
  n132 = Release Queue(queue=w23) -> ()  [unwired: 2 in, 3 out]
  n133 = xnode ("Close FPGA VI Reference")("FPGA VI Reference In"=w40, "error in"=w42) -> ("error out"=w41:errorcluster)
  n134 = Release Queue(queue=w32) -> ()  [unwired: 2 in, 3 out]
  n135 = Release Queue(queue=w28) -> ()  [unwired: 2 in, 3 out]
  n136 = flat-sequence {
    tunnel: w41 -> [w352]
    frame #0 {
      n137 = local write "Global Stop"(FALSE ("Global Stop")) -> ()
      "error out" <- w352
    }
  }
